vi "Connector Pane Lookup.vi"(10 "TermBnds":T1(array[cluster]), 11 "Pattern":u32) -> (3 "columns":cluster{"rows":u8[]}[](array[cluster]))   [LabVIEW 2019, in "Builtins.lvlib"]
doc: "Returns terminal indexes sorted into columns and rows to connect terminals left-to-right then top-to-bottom. The indexes factor in the different connector pane patterns and rotation in degrees.\n\nCreated by: Ryan Pacini"
uses:
  Builtins.lvlib
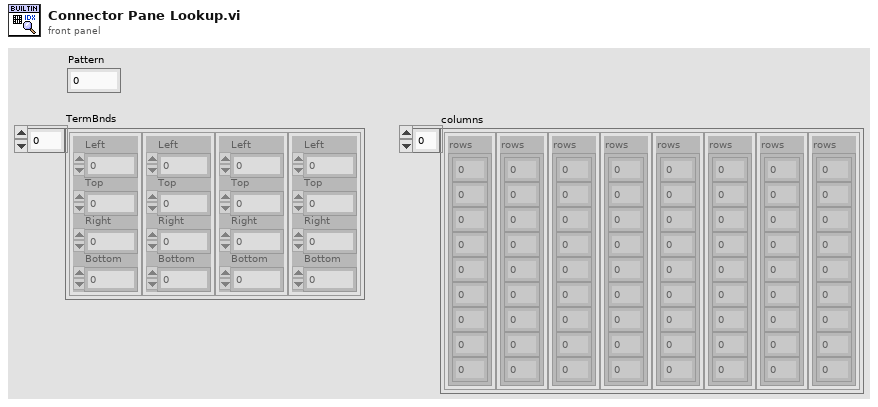
[diagram p1: front panel]
types:
  T1 = cluster{"Left":i16, "Top":i16, "Right":i16, "Bottom":i16}[]
  T2 = cluster{"pattern":u32, "rotations":cluster{"c0_term":cluster{"Left":i16, "Top":i16, "Right":i16, "Bottom":i16}, "col_idx":cluster{"row_idx":u8[]}[]}[]}[]
  T3 = cluster{"pattern":u32, "rotations":cluster{"c0_term":cluster{"Left":i16, "Top":i16, "Right":i16, "Bottom":i16}, "col_idx":cluster{"row_idx":u8[]}[]}[]}
  T4 = cluster{"c0_term":cluster{"Left":i16, "Top":i16, "Right":i16, "Bottom":i16}, "col_idx":cluster{"row_idx":u8[]}[]}[]
  T5 = cluster{"Left":i16, "Top":i16, "Right":i16, "Bottom":i16}
  T6 = cluster{"c0_term":cluster{"Left":i16, "Top":i16, "Right":i16, "Bottom":i16}, "col_idx":cluster{"row_idx":u8[]}[]}
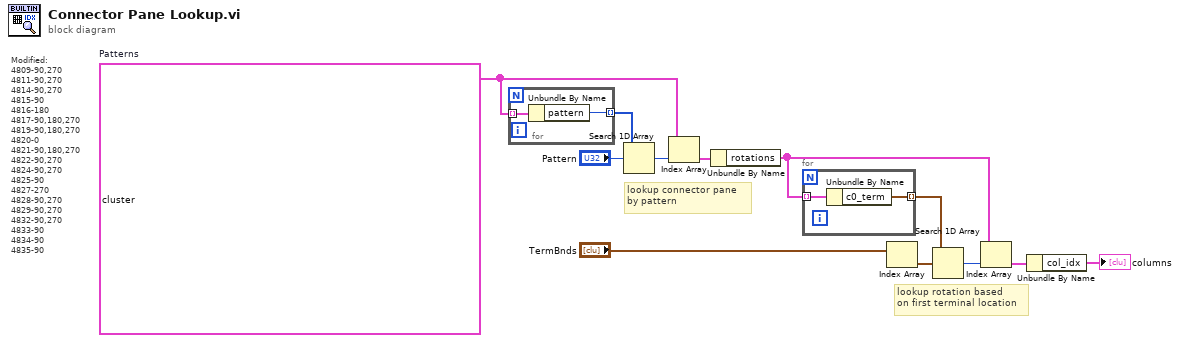
[diagram p0: block diagram]
diagram:
  w2 = T2 [{"pattern"=4800, "rotations"=[{"c0_term"={"Left"=0, "Top"=0, "Right"=32, "Bottom"=32}, "col_idx"=[{"row_idx"=[0]}]}]}, {"pattern"=4801, "rotations"=[{"c0_term"={"Left"=16, "Top"=0, "Right"=32, "Bottom"=32}, "col_idx"=[{"row_idx"=[1]}, {"row_idx"=[0]}]}, {"c0_term"={"Left"=0, "Top"=16, "Right"=32, "Bottom"=32}, "col_idx"=[{"row_idx"=[1, 0]}]}]}, {"pattern"=4802, "rotations"=[{"c0_term"={"Left"=16, "Top"=0, "Right"=32, "Bottom"=32}, "col_idx"=[{"row_idx"=[2, 1]}, {"row_idx"=[0]}]}, {"c0_term"={"Left"=0, "Top"=16, "Right"=32, "Bottom"=32}, "col_idx"=[{"row_idx"=[1, 0]}, {"row_idx"=[2]}]}, {"c0_term"={"Left"=0, "Top"=0, "Right"=16, "Bottom"=32}, "col_idx"=[{"row_idx"=[0]}, {"row_idx"=[1, 2]}]}, {"c0_term"={"Left"=0, "Top"=0, "Right"=32, "Bottom"=16}, "col_idx"=[{"row_idx"=[0, 2]}, {"row_idx"=[1]}]}]}, {"pattern"=4803, "rotations"=[{"c0_term"={"Left"=0, "Top"=21, "Right"=32, "Bottom"=32}, "col_idx"=[{"row_idx"=[2, 1, 0]}]}, {"c0_term"={"Left"=0, "Top"=0, "Right"=11, "Bottom"=32}, "col_idx"=[{"row_idx"=[0]}, {"row_idx"=[1]}, {"row_idx"=[2]}]}]}, {"pattern"=4804, "rotations"=[{"c0_term"={"Left"=16, "Top"=0, "Right"=32, "Bottom"=32}, "col_idx"=[{"row_idx"=[3, 2, 1]}, {"row_idx"=[0]}]}, {"c0_term"={"Left"=0, "Top"=16, "Right"=32, "Bottom"=32}, "col_idx"=[{"row_idx"=[1, 0]}, {"row_idx"=[2]}, {"row_idx"=[3]}]}, {"c0_term"={"Left"=0, "Top"=0, "Right"=16, "Bottom"=32}, "col_idx"=[{"row_idx"=[0]}, {"row_idx"=[1, 2, 3]}]}, {"c0_term"={"Left"=0, "Top"=0, "Right"=32, "Bottom"=16}, "col_idx"=[{"row_idx"=[0, 3]}, {"row_idx"=[2]}, {"row_idx"=[1]}]}]}, {"pattern"=4805, "rotations"=[{"c0_term"={"Left"=16, "Top"=16, "Right"=32, "Bottom"=32}, "col_idx"=[{"row_idx"=[3, 2]}, {"row_idx"=[1, 0]}]}]}, {"pattern"=4806, "rotations"=[{"c0_term"={"Left"=0, "Top"=24, "Right"=32, "Bottom"=32}, "col_idx"=[{"row_idx"=[3, 2, 1, 0]}]}, {"c0_term"={"Left"=0, "Top"=0, "Right"=8, "Bottom"=32}, "col_idx"=[{"row_idx"=[0]}, {"row_idx"=[1]}, {"row_idx"=[2]}, {"row_idx"=[3]}]}]}, {"pattern"=4807, "rotations"=[{"c0_term"={"Left"=16, "Top"=16, "Right"=32, "Bottom"=32}, "col_idx"=[{"row_idx"=[4, 3, 2]}, {"row_idx"=[1, 0]}]}, {"c0_term"={"Left"=0, "Top"=16, "Right"=16, "Bottom"=32}, "col_idx"=[{"row_idx"=[2, 0]}, {"row_idx"=[3]}, {"row_idx"=[1]}, {"row_idx"=[4]}]}, {"c0_term"={"Left"=0, "Top"=0, "Right"=16, "Bottom"=16}, "col_idx"=[{"row_idx"=[0, 1]}, {"row_idx"=[2, 3, 4]}]}, {"c0_term"={"Left"=16, "Top"=0, "Right"=32, "Bottom"=16}, "col_idx"=[{"row_idx"=[1, 4]}, {"row_idx"=[3]}, {"row_idx"=[0]}, {"row_idx"=[2]}]}]}, {"pattern"=4808, "rotations"=[{"c0_term"={"Left"=16, "Top"=0, "Right"=32, "Bottom"=32}, "col_idx"=[{"row_idx"=[4, 3, 2, 1]}, {"row_idx"=[0]}]}, {"c0_term"={"Left"=0, "Top"=16, "Right"=32, "Bottom"=32}, "col_idx"=[{"row_idx"=[1, 0]}, {"row_idx"=[2]}, {"row_idx"=[3]}, {"row_idx"=[4]}]}, {"c0_term"={"Left"=0, "Top"=0, "Right"=16, "Bottom"=32}, "col_idx"=[{"row_idx"=[0]}, {"row_idx"=[1, 2, 3, 4]}]}, {"c0_term"={"Left"=0, "Top"=0, "Right"=32, "Bottom"=16}, "col_idx"=[{"row_idx"=[0, 4]}, {"row_idx"=[3]}, {"row_idx"=[2]}, {"row_idx"=[1]}]}]}, {"pattern"=4809, "rotations"=[{"c0_term"={"Left"=16, "Top"=16, "Right"=32, "Bottom"=32}, "col_idx"=[{"row_idx"=[5, 4, 3, 2]}, {"row_idx"=[1, 0]}]}, {"c0_term"={"Left"=0, "Top"=16, "Right"=16, "Bottom"=32}, "col_idx"=[{"row_idx"=[2, 0]}, {"row_idx"=[3]}, {"row_idx"=[4]}, {"row_idx"=[5, 1]}]}, {"c0_term"={"Left"=0, "Top"=0, "Right"=16, "Bottom"=16}, "col_idx"=[{"row_idx"=[0, 1]}, {"row_idx"=[2, 3, 4, 5]}]}, {"c0_term"={"Left"=16, "Top"=0, "Right"=32, "Bottom"=16}, "col_idx"=[{"row_idx"=[1, 5]}, {"row_idx"=[4]}, {"row_idx"=[3]}, {"row_idx"=[0, 2]}]}]}, {"pattern"=4810, "rotations"=[{"c0_term"={"Left"=16, "Top"=21, "Right"=32, "Bottom"=32}, "col_idx"=[{"row_idx"=[5, 4, 3]}, {"row_idx"=[2, 1, 0]}]}, {"c0_term"={"Left"=0, "Top"=16, "Right"=11, "Bottom"=32}, "col_idx"=[{"row_idx"=[3, 0]}, {"row_idx"=[4, 1]}, {"row_idx"=[5, 2]}]}]}, {"pattern"=4811, "rotations"=[{"c0_term"={"Left"=16, "Top"=21, "Right"=32, "Bottom"=32}, "col_idx"=[{"row_idx"=[6, 5, 4, 3]}, {"row_idx"=[2, 1, 0]}]}, {"c0_term"={"Left"=0, "Top"=16, "Right"=11, "Bottom"=32}, "col_idx"=[{"row_idx"=[3, 0]}, {"row_idx"=[4, 1]}, {"row_idx"=[5]}, {"row_idx"=[6, 2]}]}, {"c0_term"={"Left"=0, "Top"=0, "Right"=16, "Bottom"=11}, "col_idx"=[{"row_idx"=[0, 1, 2]}, {"row_idx"=[3, 4, 5, 6]}]}, {"c0_term"={"Left"=21, "Top"=0, "Right"=32, "Bottom"=16}, "col_idx"=[{"row_idx"=[2, 6]}, {"row_idx"=[1, 5]}, {"row_idx"=[4]}, {"row_idx"=[0, 3]}]}]}, {"pattern"=4812, "rotations"=[{"c0_term"={"Left"=16, "Top"=24, "Right"=32, "Bottom"=32}, "col_idx"=[{"row_idx"=[7, 6, 5, 4]}, {"row_idx"=[3, 2, 1, 0]}]}, {"c0_term"={"Left"=0, "Top"=16, "Right"=8, "Bottom"=32}, "col_idx"=[{"row_idx"=[4, 0]}, {"row_idx"=[5, 1]}, {"row_idx"=[6, 2]}, {"row_idx"=[7, 3]}]}]}, {"pattern"=4813, "rotations"=[{"c0_term"={"Left"=16, "Top"=24, "Right"=32, "Bottom"=32}, "col_idx"=[{"row_idx"=[8, 7, 6, 5]}, {"row_idx"=[4]}, {"row_idx"=[3, 2, 1, 0]}]}, {"c0_term"={"Left"=0, "Top"=16, "Right"=8, "Bottom"=32}, "col_idx"=[{"row_idx"=[5, 4, 0]}, {"row_idx"=[6, 1]}, {"row_idx"=[7, 2]}, {"row_idx"=[8, 3]}]}, {"c0_term"={"Left"=0, "Top"=0, "Right"=16, "Bottom"=8}, "col_idx"=[{"row_idx"=[0, 1, 2, 3]}, {"row_idx"=[4]}, {"row_idx"=[5, 6, 7, 8]}]}, {"c0_term"={"Left"=24, "Top"=0, "Right"=32, "Bottom"=16}, "col_idx"=[{"row_idx"=[3, 4, 8]}, {"row_idx"=[2, 7]}, {"row_idx"=[1, 6]}, {"row_idx"=[0, 5]}]}]}, {"pattern"=4814, "rotations"=[{"c0_term"={"Left"=16, "Top"=24, "Right"=32, "Bottom"=32}, "col_idx"=[{"row_idx"=[9, 8, 7, 6]}, {"row_idx"=[5, 4]}, {"row_idx"=[3, 2, 1, 0]}]}, {"c0_term"={"Left"=0, "Top"=16, "Right"=8, "Bottom"=32}, "col_idx"=[{"row_idx"=[6, 4, 0]}, {"row_idx"=[7, 1]}, {"row_idx"=[8, 2]}, {"row_idx"=[9, 5, 3]}]}, {"c0_term"={"Left"=0, "Top"=0, "Right"=16, "Bottom"=8}, "col_idx"=[{"row_idx"=[0, 1, 2, 3]}, {"row_idx"=[4, 5]}, {"row_idx"=[6, 7, 8, 9]}]}, {"c0_term"={"Left"=24, "Top"=0, "Right"=32, "Bottom"=16}, "col_idx"=[{"row_idx"=[3, 5, 9]}, {"row_idx"=[2, 8]}, {"row_idx"=[1, 7]}, {"row_idx"=[0, 4, 6]}]}]}, {"pattern"=4815, "rotations"=[{"c0_term"={"Left"=24, "Top"=24, "Right"=32, "Bottom"=32}, "col_idx"=[{"row_idx"=[11, 10, 9, 8]}, {"row_idx"=[7, 6]}, {"row_idx"=[5, 4]}, {"row_idx"=[3, 2, 1, 0]}]}, {"c0_term"={"Left"=0, "Top"=24, "Right"=8, "Bottom"=32}, "col_idx"=[{"row_idx"=[8, 6, 4, 0]}, {"row_idx"=[9, 1]}, {"row_idx"=[10, 2]}, {"row_idx"=[11, 7, 5, 3]}]}]}, {"pattern"=4816, "rotations"=[{"c0_term"={"Left"=0, "Top"=0, "Right"=8, "Bottom"=11}, "col_idx"=[{"row_idx"=[0, 2, 3]}, {"row_idx"=[1, 4]}, {"row_idx"=[5]}]}, {"c0_term"={"Left"=21, "Top"=0, "Right"=32, "Bottom"=8}, "col_idx"=[{"row_idx"=[3, 4, 5]}, {"row_idx"=[2]}, {"row_idx"=[0, 1]}]}, {"c0_term"={"Left"=24, "Top"=21, "Right"=32, "Bottom"=32}, "col_idx"=[{"row_idx"=[5]}, {"row_idx"=[4, 1]}, {"row_idx"=[3, 2, 0]}]}, {"c0_term"={"Left"=0, "Top"=24, "Right"=11, "Bottom"=32}, "col_idx"=[{"row_idx"=[5, 1, 0]}, {"row_idx"=[2]}, {"row_idx"=[4, 3]}]}]}, {"pattern"=4817, "rotations"=[{"c0_term"={"Left"=0, "Top"=0, "Right"=8, "Bottom"=11}, "col_idx"=[{"row_idx"=[0, 2, 3]}, {"row_idx"=[1, 4]}, {"row_idx"=[5, 6]}]}, {"c0_term"={"Left"=21, "Top"=0, "Right"=32, "Bottom"=8}, "col_idx"=[{"row_idx"=[3, 4, 6]}, {"row_idx"=[2]}, {"row_idx"=[0, 1, 5]}]}, {"c0_term"={"Left"=24, "Top"=21, "Right"=32, "Bottom"=32}, "col_idx"=[{"row_idx"=[6, 5]}, {"row_idx"=[4, 1]}, {"row_idx"=[3, 2, 0]}]}, {"c0_term"={"Left"=0, "Top"=24, "Right"=11, "Bottom"=32}, "col_idx"=[{"row_idx"=[5, 1, 0]}, {"row_idx"=[2]}, {"row_idx"=[6, 4, 3]}]}]}, {"pattern"=4818, "rotations"=[{"c0_term"={"Left"=0, "Top"=0, "Right"=8, "Bottom"=11}, "col_idx"=[{"row_idx"=[0, 2, 3]}, {"row_idx"=[1, 4]}, {"row_idx"=[5, 6, 7]}]}, {"c0_term"={"Left"=21, "Top"=0, "Right"=32, "Bottom"=8}, "col_idx"=[{"row_idx"=[3, 4, 7]}, {"row_idx"=[2, 6]}, {"row_idx"=[0, 1, 5]}]}, {"c0_term"={"Left"=24, "Top"=21, "Right"=32, "Bottom"=32}, "col_idx"=[{"row_idx"=[7, 6, 5]}, {"row_idx"=[4, 1]}, {"row_idx"=[3, 2, 0]}]}, {"c0_term"={"Left"=0, "Top"=24, "Right"=11, "Bottom"=32}, "col_idx"=[{"row_idx"=[5, 1, 0]}, {"row_idx"=[6, 2]}, {"row_idx"=[7, 4, 3]}]}]}, {"pattern"=4819, "rotations"=[{"c0_term"={"Left"=0, "Top"=0, "Right"=8, "Bottom"=11}, "col_idx"=[{"row_idx"=[0, 2, 3]}, {"row_idx"=[1, 4]}, {"row_idx"=[5, 6, 7, 8]}]}, {"c0_term"={"Left"=21, "Top"=0, "Right"=32, "Bottom"=8}, "col_idx"=[{"row_idx"=[3, 4, 8]}, {"row_idx"=[2, 7]}, {"row_idx"=[6]}, {"row_idx"=[0, 1, 5]}]}, {"c0_term"={"Left"=24, "Top"=21, "Right"=32, "Bottom"=32}, "col_idx"=[{"row_idx"=[8, 7, 6, 5]}, {"row_idx"=[4, 1]}, {"row_idx"=[3, 2, 0]}]}, {"c0_term"={"Left"=0, "Top"=24, "Right"=11, "Bottom"=32}, "col_idx"=[{"row_idx"=[5, 1, 0]}, {"row_idx"=[6, 2]}, {"row_idx"=[7]}, {"row_idx"=[8, 4, 3]}]}]}, {"pattern"=4820, "rotations"=[{"c0_term"={"Left"=0, "Top"=0, "Right"=8, "Bottom"=11}, "col_idx"=[{"row_idx"=[0, 2, 3]}, {"row_idx"=[1, 4]}, {"row_idx"=[5, 8]}, {"row_idx"=[6, 7, 9]}]}, {"c0_term"={"Left"=21, "Top"=0, "Right"=32, "Bottom"=8}, "col_idx"=[{"row_idx"=[3, 4, 8, 9]}, {"row_idx"=[2, 7]}, {"row_idx"=[0, 1, 5, 6]}]}]}, {"pattern"=4821, "rotations"=[{"c0_term"={"Left"=0, "Top"=0, "Right"=8, "Bottom"=11}, "col_idx"=[{"row_idx"=[0, 2, 3]}, {"row_idx"=[1, 4]}, {"row_idx"=[5, 8]}, {"row_idx"=[6, 7, 9, 10]}]}, {"c0_term"={"Left"=21, "Top"=0, "Right"=32, "Bottom"=8}, "col_idx"=[{"row_idx"=[3, 4, 8, 10]}, {"row_idx"=[2, 9]}, {"row_idx"=[7]}, {"row_idx"=[0, 1, 5, 6]}]}, {"c0_term"={"Left"=24, "Top"=21, "Right"=32, "Bottom"=32}, "col_idx"=[{"row_idx"=[10, 9, 7, 6]}, {"row_idx"=[8, 5]}, {"row_idx"=[4, 1]}, {"row_idx"=[3, 2, 0]}]}, {"c0_term"={"Left"=0, "Top"=24, "Right"=11, "Bottom"=32}, "col_idx"=[{"row_idx"=[6, 5, 1, 0]}, {"row_idx"=[7, 2]}, {"row_idx"=[9]}, {"row_idx"=[10, 8, 4, 3]}]}]}, {"pattern"=4822, "rotations"=[{"c0_term"={"Left"=0, "Top"=0, "Right"=8, "Bottom"=8}, "col_idx"=[{"row_idx"=[0, 2, 3, 5]}, {"row_idx"=[1, 4]}, {"row_idx"=[6, 7, 8]}]}, {"c0_term"={"Left"=24, "Top"=0, "Right"=32, "Bottom"=8}, "col_idx"=[{"row_idx"=[5, 4, 8]}, {"row_idx"=[3, 7]}, {"row_idx"=[2]}, {"row_idx"=[0, 1, 6]}]}, {"c0_term"={"Left"=24, "Top"=24, "Right"=32, "Bottom"=32}, "col_idx"=[{"row_idx"=[8, 7, 6]}, {"row_idx"=[4, 1]}, {"row_idx"=[5, 3, 2, 0]}]}, {"c0_term"={"Left"=0, "Top"=24, "Right"=8, "Bottom"=32}, "col_idx"=[{"row_idx"=[6, 1, 0]}, {"row_idx"=[7, 2]}, {"row_idx"=[3]}, {"row_idx"=[8, 4, 5]}]}]}, {"pattern"=4823, "rotations"=[{"c0_term"={"Left"=0, "Top"=0, "Right"=8, "Bottom"=8}, "col_idx"=[{"row_idx"=[0, 1, 2, 3]}, {"row_idx"=[4]}, {"row_idx"=[5]}]}, {"c0_term"={"Left"=24, "Top"=0, "Right"=32, "Bottom"=8}, "col_idx"=[{"row_idx"=[3, 4, 5]}, {"row_idx"=[2]}, {"row_idx"=[1]}, {"row_idx"=[0]}]}, {"c0_term"={"Left"=24, "Top"=24, "Right"=32, "Bottom"=32}, "col_idx"=[{"row_idx"=[5]}, {"row_idx"=[4]}, {"row_idx"=[3, 2, 1, 0]}]}, {"c0_term"={"Left"=0, "Top"=24, "Right"=8, "Bottom"=32}, "col_idx"=[{"row_idx"=[5, 4, 0]}, {"row_idx"=[1]}, {"row_idx"=[2]}, {"row_idx"=[3]}]}]}, {"pattern"=4824, "rotations"=[{"c0_term"={"Left"=0, "Top"=0, "Right"=8, "Bottom"=8}, "col_idx"=[{"row_idx"=[0, 1, 2, 3]}, {"row_idx"=[4]}, {"row_idx"=[5, 6]}]}, {"c0_term"={"Left"=24, "Top"=0, "Right"=32, "Bottom"=8}, "col_idx"=[{"row_idx"=[3, 4, 6]}, {"row_idx"=[2]}, {"row_idx"=[1]}, {"row_idx"=[0, 5]}]}, {"c0_term"={"Left"=24, "Top"=24, "Right"=32, "Bottom"=32}, "col_idx"=[{"row_idx"=[6, 5]}, {"row_idx"=[4]}, {"row_idx"=[3, 2, 1, 0]}]}, {"c0_term"={"Left"=0, "Top"=24, "Right"=8, "Bottom"=32}, "col_idx"=[{"row_idx"=[5, 4, 0]}, {"row_idx"=[1]}, {"row_idx"=[2]}, {"row_idx"=[6, 3]}]}]}, {"pattern"=4825, "rotations"=[{"c0_term"={"Left"=0, "Top"=0, "Right"=8, "Bottom"=8}, "col_idx"=[{"row_idx"=[0, 1, 2, 3]}, {"row_idx"=[4]}, {"row_idx"=[5, 6, 7]}]}, {"c0_term"={"Left"=24, "Top"=0, "Right"=32, "Bottom"=8}, "col_idx"=[{"row_idx"=[3, 4, 7]}, {"row_idx"=[2, 6]}, {"row_idx"=[1]}, {"row_idx"=[0, 5]}]}, {"c0_term"={"Left"=24, "Top"=24, "Right"=32, "Bottom"=32}, "col_idx"=[{"row_idx"=[7, 6, 5]}, {"row_idx"=[4]}, {"row_idx"=[3, 2, 1, 0]}]}, {"c0_term"={"Left"=0, "Top"=24, "Right"=8, "Bottom"=32}, "col_idx"=[{"row_idx"=[5, 4, 0]}, {"row_idx"=[6, 1]}, {"row_idx"=[2]}, {"row_idx"=[7, 3]}]}]}, {"pattern"=4826, "rotations"=[{"c0_term"={"Left"=24, "Top"=24, "Right"=32, "Bottom"=32}, "col_idx"=[{"row_idx"=[9, 8, 7, 6]}, {"row_idx"=[5]}, {"row_idx"=[4]}, {"row_idx"=[3, 2, 1, 0]}]}, {"c0_term"={"Left"=0, "Top"=24, "Right"=8, "Bottom"=32}, "col_idx"=[{"row_idx"=[6, 5, 4, 0]}, {"row_idx"=[7, 1]}, {"row_idx"=[8, 2]}, {"row_idx"=[9, 3]}]}]}, {"pattern"=4827, "rotations"=[{"c0_term"={"Left"=16, "Top"=0, "Right"=32, "Bottom"=32}, "col_idx"=[{"row_idx"=[6, 5, 4, 3]}, {"row_idx"=[2, 1]}, {"row_idx"=[0]}]}, {"c0_term"={"Left"=0, "Top"=16, "Right"=32, "Bottom"=32}, "col_idx"=[{"row_idx"=[3, 1, 0]}, {"row_idx"=[4]}, {"row_idx"=[5]}, {"row_idx"=[6, 2]}]}, {"c0_term"={"Left"=0, "Top"=0, "Right"=16, "Bottom"=32}, "col_idx"=[{"row_idx"=[0]}, {"row_idx"=[1, 2]}, {"row_idx"=[3, 4, 5, 6]}]}, {"c0_term"={"Left"=0, "Top"=0, "Right"=32, "Bottom"=16}, "col_idx"=[{"row_idx"=[0, 2, 6]}, {"row_idx"=[5]}, {"row_idx"=[4]}, {"row_idx"=[1, 3]}]}]}, {"pattern"=4828, "rotations"=[{"c0_term"={"Left"=16, "Top"=16, "Right"=32, "Bottom"=32}, "col_idx"=[{"row_idx"=[7, 6, 5, 4]}, {"row_idx"=[3, 2]}, {"row_idx"=[1, 0]}]}, {"c0_term"={"Left"=0, "Top"=16, "Right"=16, "Bottom"=32}, "col_idx"=[{"row_idx"=[4, 2, 0]}, {"row_idx"=[5]}, {"row_idx"=[6]}, {"row_idx"=[7, 3, 1]}]}, {"c0_term"={"Left"=0, "Top"=0, "Right"=16, "Bottom"=16}, "col_idx"=[{"row_idx"=[0, 1]}, {"row_idx"=[2, 3]}, {"row_idx"=[4, 5, 6, 7]}]}, {"c0_term"={"Left"=16, "Top"=0, "Right"=32, "Bottom"=16}, "col_idx"=[{"row_idx"=[1, 3, 7]}, {"row_idx"=[6]}, {"row_idx"=[5]}, {"row_idx"=[0, 2, 4]}]}]}, {"pattern"=4829, "rotations"=[{"c0_term"={"Left"=24, "Top"=24, "Right"=32, "Bottom"=32}, "col_idx"=[{"row_idx"=[10, 9, 8, 7]}, {"row_idx"=[6, 5]}, {"row_idx"=[4]}, {"row_idx"=[3, 2, 1, 0]}]}, {"c0_term"={"Left"=0, "Top"=24, "Right"=8, "Bottom"=32}, "col_idx"=[{"row_idx"=[7, 5, 4, 0]}, {"row_idx"=[8, 1]}, {"row_idx"=[9, 2]}, {"row_idx"=[10, 6, 3]}]}, {"c0_term"={"Left"=0, "Top"=0, "Right"=8, "Bottom"=8}, "col_idx"=[{"row_idx"=[0, 1, 2, 3]}, {"row_idx"=[4]}, {"row_idx"=[5, 6]}, {"row_idx"=[7, 8, 9, 10]}]}, {"c0_term"={"Left"=24, "Top"=0, "Right"=32, "Bottom"=8}, "col_idx"=[{"row_idx"=[3, 4, 6, 10]}, {"row_idx"=[2, 9]}, {"row_idx"=[1, 8]}, {"row_idx"=[0, 5, 7]}]}]}, {"pattern"=4830, "rotations"=[{"c0_term"={"Left"=21, "Top"=0, "Right"=32, "Bottom"=32}, "col_idx"=[{"row_idx"=[3, 2]}, {"row_idx"=[1]}, {"row_idx"=[0]}]}, {"c0_term"={"Left"=0, "Top"=21, "Right"=32, "Bottom"=32}, "col_idx"=[{"row_idx"=[2, 1, 0]}, {"row_idx"=[3]}]}, {"c0_term"={"Left"=0, "Top"=0, "Right"=11, "Bottom"=32}, "col_idx"=[{"row_idx"=[0]}, {"row_idx"=[1]}, {"row_idx"=[2, 3]}]}, {"c0_term"={"Left"=0, "Top"=0, "Right"=32, "Bottom"=11}, "col_idx"=[{"row_idx"=[0, 1, 3]}, {"row_idx"=[2]}]}]}, {"pattern"=4831, "rotations"=[{"c0_term"={"Left"=21, "Top"=0, "Right"=32, "Bottom"=32}, "col_idx"=[{"row_idx"=[4, 3, 2]}, {"row_idx"=[1]}, {"row_idx"=[0]}]}, {"c0_term"={"Left"=0, "Top"=21, "Right"=32, "Bottom"=32}, "col_idx"=[{"row_idx"=[2, 1, 0]}, {"row_idx"=[3]}, {"row_idx"=[4]}]}, {"c0_term"={"Left"=0, "Top"=0, "Right"=11, "Bottom"=32}, "col_idx"=[{"row_idx"=[0]}, {"row_idx"=[1]}, {"row_idx"=[2, 3, 4]}]}, {"c0_term"={"Left"=0, "Top"=0, "Right"=32, "Bottom"=11}, "col_idx"=[{"row_idx"=[0, 1, 4]}, {"row_idx"=[3]}, {"row_idx"=[2]}]}]}, {"pattern"=4832, "rotations"=[{"c0_term"={"Left"=21, "Top"=16, "Right"=32, "Bottom"=32}, "col_idx"=[{"row_idx"=[5, 4, 3]}, {"row_idx"=[2]}, {"row_idx"=[1, 0]}]}, {"c0_term"={"Left"=0, "Top"=21, "Right"=16, "Bottom"=32}, "col_idx"=[{"row_idx"=[3, 2, 0]}, {"row_idx"=[4]}, {"row_idx"=[5, 1]}]}, {"c0_term"={"Left"=0, "Top"=0, "Right"=11, "Bottom"=16}, "col_idx"=[{"row_idx"=[0, 1]}, {"row_idx"=[2]}, {"row_idx"=[3, 4, 5]}]}, {"c0_term"={"Left"=16, "Top"=0, "Right"=32, "Bottom"=11}, "col_idx"=[{"row_idx"=[1, 2, 5]}, {"row_idx"=[4]}, {"row_idx"=[0, 3]}]}]}, {"pattern"=4833, "rotations"=[{"c0_term"={"Left"=0, "Top"=0, "Right"=7, "Bottom"=7}, "col_idx"=[{"row_idx"=[0, 5, 7, 9, 11]}, {"row_idx"=[1, 12]}, {"row_idx"=[2, 13]}, {"row_idx"=[3, 14]}, {"row_idx"=[4, 6, 8, 10, 15]}]}, {"c0_term"={"Left"=25, "Top"=0, "Right"=32, "Bottom"=7}, "col_idx"=[{"row_idx"=[11, 12, 13, 14, 15]}, {"row_idx"=[9, 10]}, {"row_idx"=[7, 8]}, {"row_idx"=[5, 6]}, {"row_idx"=[0, 1, 2, 3, 4]}]}]}, {"pattern"=4834, "rotations"=[{"c0_term"={"Left"=0, "Top"=0, "Right"=6, "Bottom"=6}, "col_idx"=[{"row_idx"=[0, 1, 2, 3, 4, 5]}, {"row_idx"=[6, 7]}, {"row_idx"=[8, 9]}, {"row_idx"=[10, 11]}, {"row_idx"=[12, 13]}, {"row_idx"=[14, 15, 16, 17, 18, 19]}]}, {"c0_term"={"Left"=26, "Top"=0, "Right"=32, "Bottom"=6}, "col_idx"=[{"row_idx"=[5, 7, 9, 11, 13, 19]}, {"row_idx"=[4, 18]}, {"row_idx"=[3, 17]}, {"row_idx"=[2, 16]}, {"row_idx"=[1, 15]}, {"row_idx"=[0, 6, 8, 10, 12, 14]}]}]}, {"pattern"=4835, "rotations"=[{"c0_term"={"Left"=0, "Top"=0, "Right"=4, "Bottom"=4}, "col_idx"=[{"row_idx"=[0, 1, 2, 3, 4, 5, 6, 7]}, {"row_idx"=[8, 9]}, {"row_idx"=[10, 11]}, {"row_idx"=[12, 13]}, {"row_idx"=[14, 15]}, {"row_idx"=[16, 17]}, {"row_idx"=[18, 19]}, {"row_idx"=[20, 21, 22, 23, 24, 25, 26, 27]}]}, {"c0_term"={"Left"=28, "Top"=0, "Right"=32, "Bottom"=4}, "col_idx"=[{"row_idx"=[7, 9, 11, 13, 15, 17, 19, 27]}, {"row_idx"=[6, 26]}, {"row_idx"=[5, 25]}, {"row_idx"=[4, 24]}, {"row_idx"=[3, 23]}, {"row_idx"=[2, 22]}, {"row_idx"=[1, 21]}, {"row_idx"=[0, 8, 10, 12, 14, 16, 18, 20]}]}]}]  # Patterns
  # "lookup rotation based\non first terminal location"
  # "lookup connector pane\nby pattern"
  # "Modified:\n4809-90,270\n4811-90,270\n4814-90,270\n4815-90\n4816-180\n4817-90,180,270\n4819-90,180,270\n4820-0\n4821-90,180,270\n4822-90,270\n4824-90,270\n4825-90\n4827-270\n4828-90,270\n4829-90,270\n4832-90,270\n4833-90\n4834-90\n4835-90"
  n1 = for {
    tunnel: w2 -> [w14] mode=indexing
    tunnel: [w13] -> w11 mode=indexing
    n2 = Unbundle By Name(w14) -> ("pattern"=w13:u32)
  }
  n3 = Search 1D Array(1D array=w11, element="Pattern") -> (index of element=w9:i32)  [unwired: 1 in]
  n4 = Index Array(array=w2, index=w9) -> (element=w8:T3)
  n5 = Unbundle By Name(w8) -> ("rotations"=w5:T4)
  n6 = for {
    tunnel: w5 -> [w16] mode=indexing
    tunnel: [w15] -> w6 mode=indexing
    n7 = Unbundle By Name(w16) -> ("c0_term"=w15:T5)
  }
  n8 = Index Array(array="TermBnds") -> (element=w3:T5)  [unwired: 1 in]
  n9 = Search 1D Array(1D array=w6, element=w3) -> (index of element=w1:i32)  [unwired: 1 in]
  n10 = Index Array(array=w5, index=w1) -> (element=w7:T6)
  n11 = Unbundle By Name(w7) -> ("col_idx"=→"columns":cluster{"row_idx":u8[]}[])
